vi "Pass.vi"(7 "Description":string, 8 "error in (no error)":errorcluster, 9 "Message":string, 11 "LUnit Test Case In":refnum<class "LUnit Test Case V2.lvclass">) -> (0 "error out":errorcluster, 3 "LUnit Test Case Out":refnum<class "LUnit Test Case V2.lvclass">)   [LabVIEW 2020, in "LUnit Test Case V2.lvclass"]
doc: "Generates a pass result for the calling test method. A description and message may be provided."
uses:
  LUnit Test Case V2.lvclass
  Framework/Result Types/Assertion Result/Assertion Result.ctl
  Framework/Result Types/Assertion Result/Public/TypeDefs/Status.ctl
  Framework/Result Types/Assertion Result/Public/TypeDefs/Assertion Type.ctl
  LUnit Test Case V2.lvclass/LUnit Test Case V2.ctl
  Framework/Result Types/Assertion Result/Assertion Result.lvlib
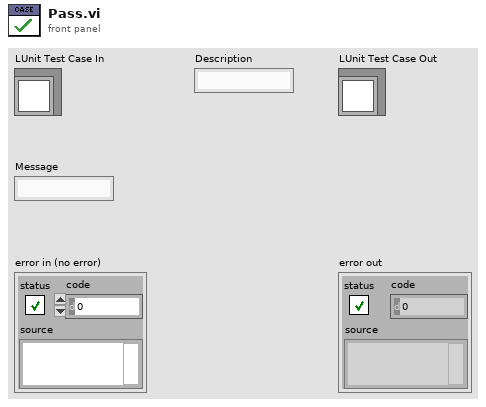
[diagram p1: front panel]
types:
  T1 = typedef "Assertion Result.lvlib/Assertion Result.ctl" = cluster{"Status":T2, "Message":string, "Description":string, "Assertion Type":T3}
  T2 = typedef "Assertion Result.lvlib/Status.ctl" = enum16{"Pass", "Fail", "Error", "Skipped", "Setup Error", "Broken", "Teardown Error"}
  T3 = typedef "Assertion Result.lvlib/Assertion Type.ctl" = enum16{"None", "Pass", "Fail", "Skip", "Pass if Equal", "Fail if Equal", "Pass if Error", "Fail if Error", "Pass if", "Fail if"}
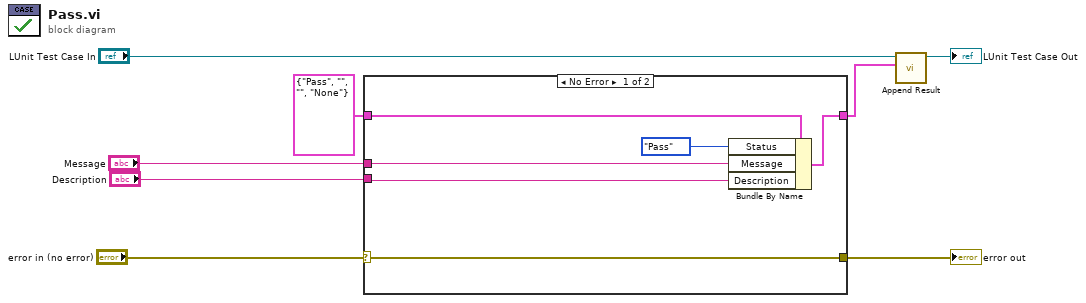
[diagram p0: block diagram]
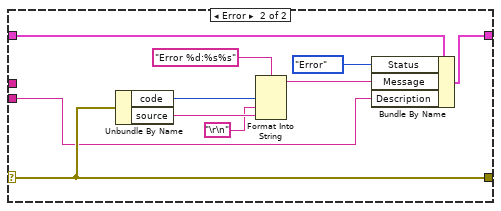
[diagram p2: hidden frame]
diagram:
  n1 = case shown="No Error" "error in (no error)" {
    selector: "error in (no error)" -> [w12 w20]
    tunnel: T1 {"Status"=enum."Pass", "Message"="", "Description"="", "Assertion Type"=enum."None"} ("Temporary Assertion Result") -> [w14 w16]
    tunnel: [w13 w17] -> w1
    tunnel: [w12 w20] -> w6
    tunnel: "Message" -> [w11 _]
    tunnel: "Description" -> [w9 w15]
    frame No Error {
      n2 = Bundle By Name(cluster=w14, "Status"=Status."Pass", "Message"=w11, "Description"=w9) -> (w13:T1)
    }
    frame Error {
      n3 = Unbundle By Name(w20) -> ("code"=w24:i32, "source"=w22:string)
      n4 = Format Into String(format string="Error %d:%s%s", w24, "\r\n", w22) -> (resulting string=w23:string)  [unwired: 2 in, 1 out]
      n5 = Bundle By Name(cluster=w16, "Status"=Status."Error", "Message"=w23, "Description"=w15) -> (w17:T1)
    }
  }
  "error out" <- w6
  n6 = call "Append Result.vi"("Temporary Assertion Result"=w1, "LUnit Test Case V2 in"="LUnit Test Case In") -> ("LUnit Test Case V2 out"=→"LUnit Test Case Out":refnum<class "LUnit Test Case V2.lvclass">)  [unwired: 9 in]
